vi "SyncLoop.vi"(8 "error in (no error)":errorcluster, 11 "PXI_MultiTrig in":refnum<class "PXI_MultiTrig.lvclass">) -> (0 "error out":errorcluster, 1 "Locked":bool, 2 "Time Ref Offset (ns)":dbl format="%#_12f", 3 "PXI_MultiTrig out":refnum<class "PXI_MultiTrig.lvclass">, 4 "LostLock":bool, 6 "ObtainLock":bool)   [LabVIEW 2018, in "SyncPlugins.lvlib" / "PXI_MultiTrig.lvclass"]
uses:
  PXI_MultiTrig.lvclass
  X:/Projects/NistPluggableModules/dev/NistPluggableModules/Sync/SyncPlugins/SyncPluginBase/SyncPluginBase.lvclass
  Typedefs/clClocks.ctl
  SyncPluginBase/SyncPluginBase.lvclass/SyncPluginBase.ctl
  PXI_MultiTrig.lvclass/PXI_MultiTrig.ctl
  SyncPluginBase/Accessors/Write Locked.vi
  SyncPluginBase/Accessors/Write LostLock.vi
  Accessors/Read SyncWindowsClock.vi
  Accessors/Read RefClkSession.vi
  Accessors/Read SysRef.vi
  SyncPluginBase/Accessors/Write PPSTime.vi
  Accessors/Read Clocks.vi
  SyncPluginBase/Accessors/Read Run.vi
  Accessors/Read TimingSession.vi
  SyncPluginBase/Accessors/Read Initiated.vi
  SyncPluginBase/Accessors/Read Locked.vi
  <instrlib>/niSync/niSync.llb/niSync Read Trigger Time Stamp (Single).vi
  <resource>/objmgr/niMIDebugSession.rc
  SyncPluginBase/SyncPluginBase.lvclass
panel:
  out "Time:Current time":timestamp
  out "Clocks":T1[](array[typedef])
  out "RefClk Present":bool
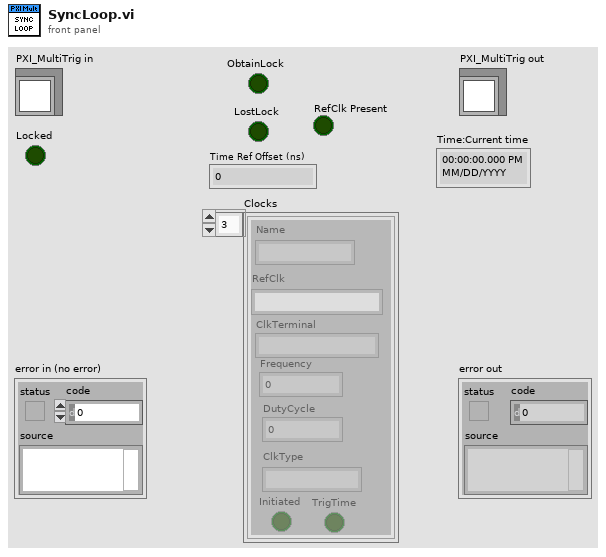
[diagram p1: front panel]
types:
  T1 = typedef "SyncPlugins.lvlib/PXI_MultiTrig.lvclass/clClocks.ctl" = cluster{"Name":string, "RefClk":string, "ClkTerminal":string, "Frequency":dbl, "DutyCycle":dbl, "ClkType":string, "Initiated":bool, "TrigTime":bool}
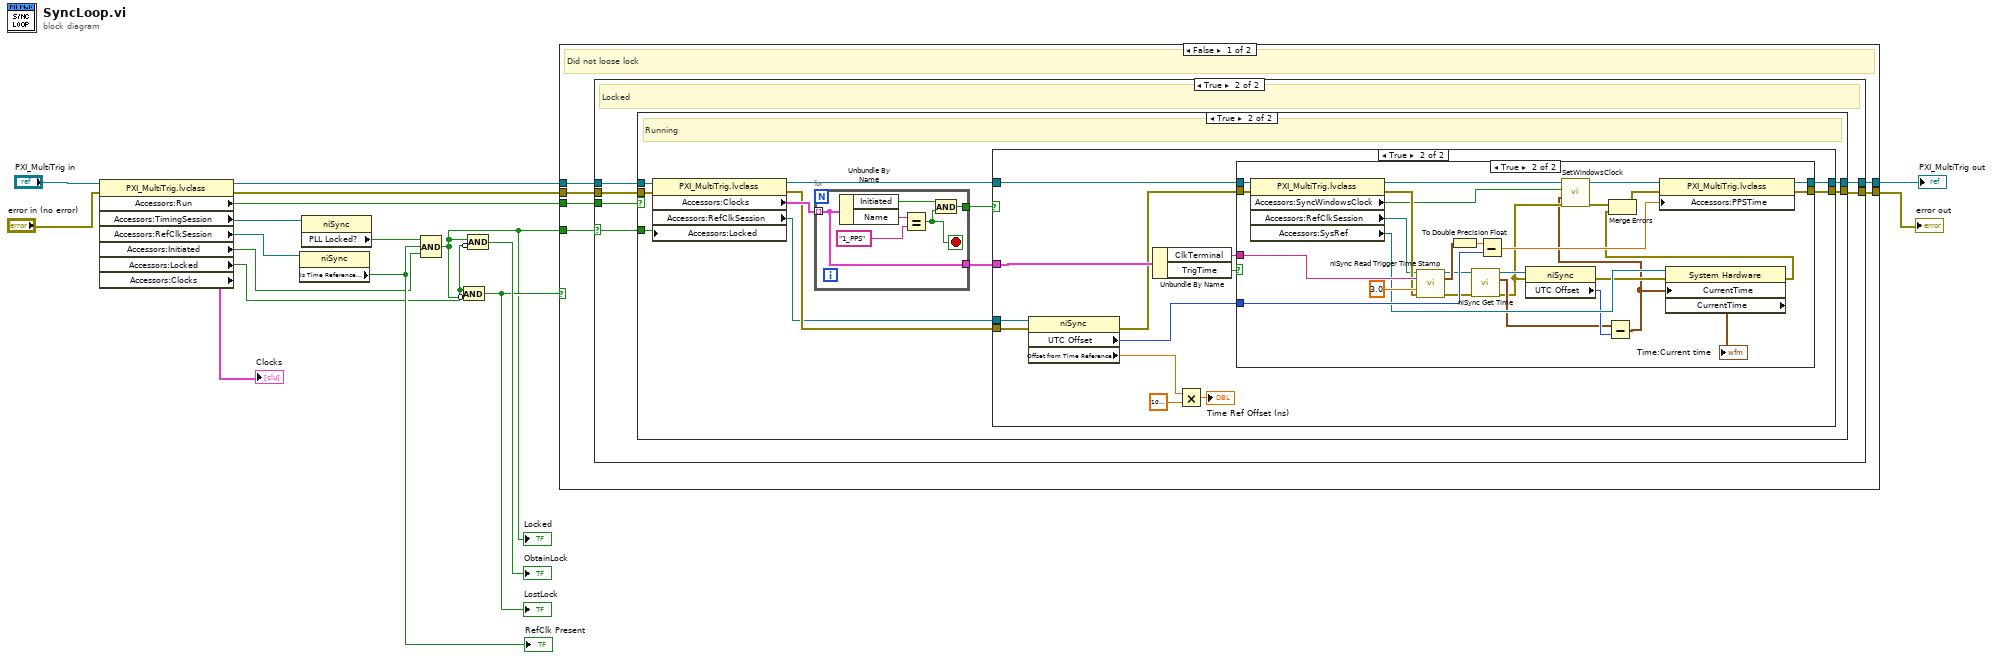
[diagram p0: block diagram]
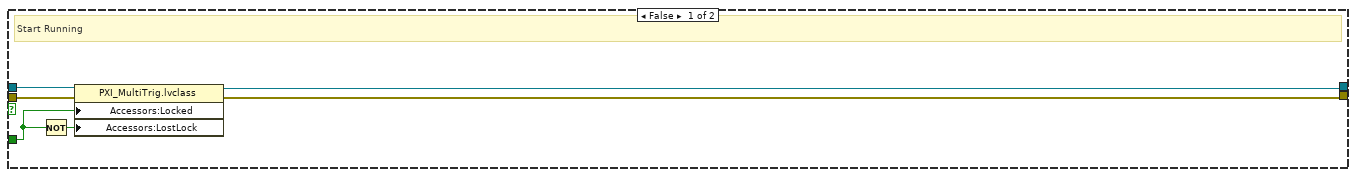
[diagram p3: hidden frame]
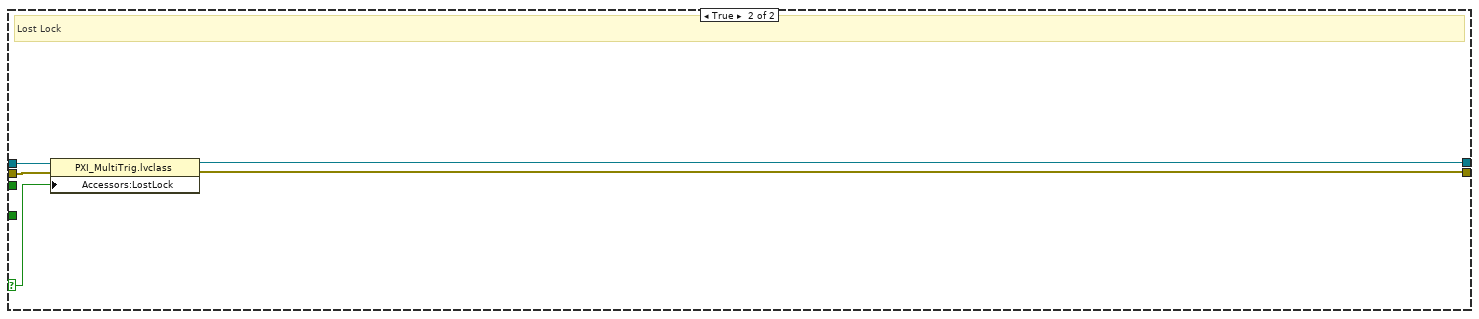
[diagram p6: hidden frame]
diagram:
  n1 = property class="PXI_MultiTrig.lvclass"(reference="PXI_MultiTrig in", error in="error in (no error)") -> (reference out=w11:refnum<class "PXI_MultiTrig.lvclass">, error out=w9:errorcluster, "Accessors:Run"=w8:bool, "Accessors:TimingSession"=w13:refnum<k15>, "Accessors:RefClkSession"=w4:refnum<k15>, "Accessors:Initiated"=w2:bool, "Accessors:Locked"=w3:bool, "Accessors:Clocks"=→"Clocks":T1[])
  n2 = property class="niSync"(reference=w4) -> ("Is Time Reference Present"=w5:bool)  [unwired: 1 in, 2 out]
  "RefClk Present" <- w5
  n3 = property class="niSync"(reference=w13) -> ("PLL Locked?"=w7:bool)  [unwired: 1 in, 2 out]
  n4 = Compound Arithmetic op=AND(w7, w5, w2) -> (w6:bool)
  "Locked" <- w6
  n5 = Compound Arithmetic op=AND(w3, invert w6) -> (w10:bool)
  "LostLock" <- w10
  n6 = Compound Arithmetic op=AND(w6, invert w3) -> (→"ObtainLock":bool)
  n7 = case shown="False" w10 {
    selector: w10 -> [_ w102]
    tunnel: [w23 w101] -> w17
    tunnel: [w18 w100] -> w16
    tunnel: w11 -> [w21 w104]
    tunnel: w9 -> [w20 w103]
    tunnel: w6 -> [w22 _]
    tunnel: w8 -> [w19 _]
    frame False {
      # "Did not loose lock"
      n8 = case shown="True" w22 {
        selector: w22 -> [_ w26]
        tunnel: [w25 w31] -> w23
        tunnel: w21 -> [w25 w30]
        tunnel: w20 -> [w24 w29]
        tunnel: w19 -> [_ w28]
        tunnel: [w24 w27] -> w18
        frame False {
          # "Not yet locked"
        }
        frame True {
          # "Locked"
          n9 = case shown="True" w28 {
            tunnel: [w35 w44] -> w31
            tunnel: w30 -> [w37 w48]
            tunnel: w29 -> [w36 w47]
            tunnel: [w34 w41] -> w27
            tunnel: w26 -> [w33 w40]
            frame False {
              # "Start Running"
              n10 = Not(x=w33) -> (.not. x?=w32:bool)
              n11 = property class="PXI_MultiTrig.lvclass"(reference=w37, error in=w36, "Accessors:Locked"=w33, "Accessors:LostLock"=w32) -> (reference out=w35:refnum<class "PXI_MultiTrig.lvclass">, error out=w34:errorcluster)
            }
            frame True {
              # "Running"
              n12 = property class="PXI_MultiTrig.lvclass"(reference=w48, error in=w47, "Accessors:Locked"=w40) -> (reference out=w45:refnum<class "PXI_MultiTrig.lvclass">, error out=w39:errorcluster, "Accessors:Clocks"=w46:T1[], "Accessors:RefClkSession"=w38:refnum<k15>)
              n13 = for {
                tunnel: w46 -> [w97] mode=indexing
                tunnel: [w97] -> w43
                tunnel: [w94] -> w42
                stop <- w96 stop-if-true
                n14 = Unbundle By Name(w97) -> ("Initiated"=w95:bool, "Name"=w99:string)
                n15 = Equal?(x=w99, y="1_PPS") -> (x = y?=w96:bool)
                n16 = And(x=w95, y=w96) -> (x .and. y?=w94:bool)
              }
              n17 = case shown="True" w42 {
                tunnel: w45 -> [w50 w63]
                tunnel: [w50 w62] -> w44
                tunnel: w43 -> [_ w61]
                tunnel: [w49 w59] -> w41
                tunnel: w39 -> [w49 w57]
                tunnel: w38 -> [_ w55]
                frame False {
                }
                frame True {
                  n18 = property class="niSync"(reference=w55, error in=w57) -> (error out=w56:errorcluster, "UTC Offset"=w54:i32, "Offset from Time Reference"=w53:dbl)  [unwired: 1 out]
                  n19 = Unbundle By Name(w61) -> ("ClkTerminal"=w60:string, "TrigTime"=w58:bool)
                  n20 = Multiply(x=w53, y=1000000000.0) -> (x*y=→"Time Ref Offset (ns)":dbl)
                  n21 = case shown="True" w58 {
                    tunnel: w63 -> [w65 w93]
                    tunnel: [w65 w92] -> w62
                    tunnel: w60 -> [_ w91]
                    tunnel: w54 -> [_ w87]
                    tunnel: w56 -> [w64 w85]
                    tunnel: [w64 w80] -> w59
                    frame False {
                    }
                    frame True {
                      n22 = property class="PXI_MultiTrig.lvclass"(reference=w93, error in=w85) -> (reference out=w76:refnum<class "PXI_MultiTrig.lvclass">, error out=w84:errorcluster, "Accessors:SyncWindowsClock"=w72:bool, "Accessors:RefClkSession"=w74:refnum<k15>, "Accessors:SysRef"=w81:refnum<k20>)
                      n23 = call-poly <instrlib>:"niSync Read Trigger Time Stamp.vi"("instrument handle"=w74, "terminal"=w91, "timeout"=3.0, "error in (no error)"=w84) -> ("instrument handle out"=w83:refnum<k15>, "time stamp out"=w89:timestamp, "error out"=w82:errorcluster)  [unwired: 8 in, 1 out]
                      n24 = To Double Precision Float(number=w89) -> (double precision float=w88:dbl)
                      n25 = call <instrlib>:"niSync Get Time.vi"("error in (no error)"=w82, "instrument handle"=w83) -> ("error out"=w70:errorcluster, "time"=w73:timestamp, "instrument handle out"=w78:refnum<k15>)  [unwired: 5 in]
                      n26 = Subtract(x=w88, y=w87) -> (x-y=w86:dbl)
                      n27 = property class="niSync"(reference=w78, error in=w70) -> (error out=w71:errorcluster, "UTC Offset"=w77:i32)  [unwired: 1 out]
                      n28 = Subtract(x=w73, y=w77) -> (x-y=w66:timestamp)
                      n29 = call "SetWindowsClock.vi"("error in (no error)"=w70, "time stamp"=w66, "SyncWinClk"=w72, "SyncPluginBase in"=w76) -> ("error out"=w69:errorcluster, "SyncPluginBase out"=w75:refnum<class "PXI_MultiTrig.lvclass">)  [unwired: 6 in]
                      n30 = property class="System Hardware"(reference=w81, error in=w71, "CurrentTime"=w66) -> (error out=w67:errorcluster, "CurrentTime"=→"Time:Current time":timestamp)  [unwired: 1 out]
                      n31 = Merge Errors(w69, w67) -> (w68:errorcluster)
                      n32 = property class="PXI_MultiTrig.lvclass"(reference=w75, error in=w68, "Accessors:PPSTime"=w86) -> (reference out=w92:refnum<class "PXI_MultiTrig.lvclass">, error out=w80:errorcluster)
                    }
                  }
                }
              }
            }
          }
        }
      }
    }
    frame True {
      # "Lost Lock"
      n33 = property class="PXI_MultiTrig.lvclass"(reference=w104, error in=w103, "Accessors:LostLock"=w102) -> (reference out=w101:refnum<class "PXI_MultiTrig.lvclass">, error out=w100:errorcluster)
    }
  }
  "error out" <- w16
  "PXI_MultiTrig out" <- w17
